vi "OAT Order Magnitude and Phase.vi"   [LabVIEW 2017, in "SoundVib_OrderTracking.lvlib"]
doc: "Computes the magnitudes and phases of designated orders in an even-angle signal. Use this VI to track particular orders specified by <B>orders to compute</B>. Wire data to the <B>even-angle signal</B> input to determine the polymorphic instance to use or manually select the instance."
uses:
  <vilib>/addons/Sound and Vibration/Order Analysis/Resample Order Tracking/SoundVib_OrderTracking.lvlib
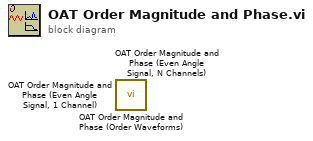
[diagram p0: block diagram]
diagram:
  n1 = call <vilib>:"OAT Order Magnitude and Phase (Order Waveforms).vi"() -> ()  [unwired: 10 in, 6 out]
  n2 = call <vilib>:"OAT Order Magnitude and Phase (Even Angle Signal, N Channels).vi"() -> ()  [unwired: 10 in, 6 out]
  n3 = call <vilib>:"OAT Order Magnitude and Phase (Even Angle Signal, 1 Channel).vi"() -> ()  [unwired: 10 in, 6 out]
